vi "Write Read.vi"(8 "error in (no error)":errorcluster, 10 "Write String":string, 11 "VISA resource name":refnum<visa-resource-name>) -> (0 "error out":errorcluster, 2 "Read Response":string, 3 "VISA resource name out":refnum<visa-resource-name>)   [LabVIEW 2023, in "Fluke Molbox 1 Plus.lvlib"]
doc: "Special write and read VI that is used for almost all VI's. Required for configures because the instrument response to a configure command is stored in the buffer until a read is performed. Therefore, in order to keep the buffer clear, there will always be a write accompanied by a read."
uses:
  Fluke Molbox 1 Plus.lvlib
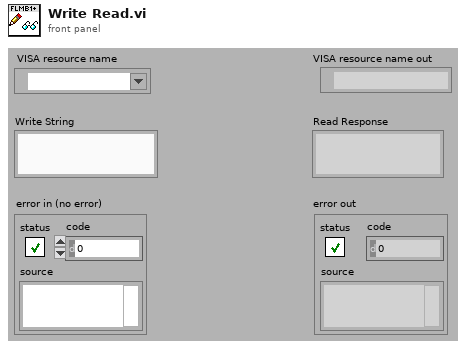
[diagram p1: front panel]
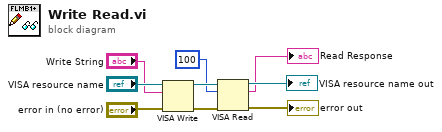
[diagram p0: block diagram]
diagram:
  n1 = VISA Write(VISA resource name="VISA resource name", write buffer="Write String", error in (no error)="error in (no error)") -> (VISA resource name out=w8:refnum<visa-resource-name>, error out=w9:errorcluster)  [unwired: 1 out]
  n2 = VISA Read(VISA resource name=w8, byte count=u32 100, error in (no error)=w9) -> (VISA resource name out=→"VISA resource name out":refnum<visa-resource-name>, read buffer=→"Read Response":string, error out=→"error out":errorcluster)  [unwired: 1 out]
